vi "get errno pointer for calling thread.vi"(8 "error in (no error)":errorcluster) -> (0 "error out":errorcluster, 3 "errno pointer":u64 format="0x%016x")   [LabVIEW 2013, in "Linux Errno.lvlib"]
uses:
  Linux Errno.lvlib
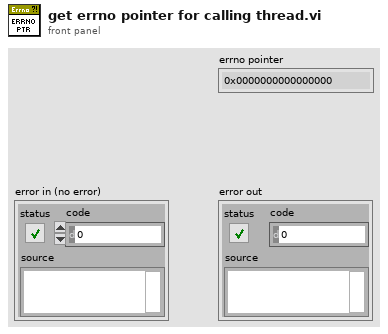
[diagram p1: front panel]
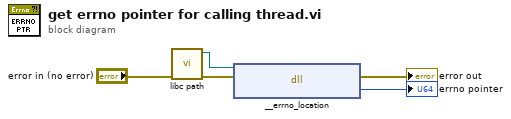
[diagram p0: block diagram]
diagram:
  n1 = call "libc path.vi"("error in (no error)"="error in (no error)") -> ("error out"=w2:errorcluster, "path to library"=w1:path)  [unwired: 9 in]
  n2 = dll-call lib="libc.so.6" fn="__errno_location"(path in=w1, error in=w2) -> (error out=→"error out":errorcluster, "return type"=→"errno pointer":u64)  [unwired: 1 in, 1 out]
